vi "规范时间戳.vi"(11 "字符串":string) -> (3 "result string":string)   [LabVIEW 2016, in "数据传输系统-04.lvlib"]
panel:
  out "输出 1":timestamp
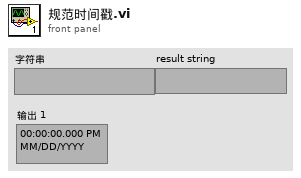
[diagram p1: front panel]
types:
  T1 = typedef "LVDateTimeRec.ctl" = cluster{"秒数的小数部分":dbl, "秒":i32, "分":i32, "时":i32, "日":i32, "月":i32, "年":i32, "天数（周）":i32, "天数（年）":i32, "DST":i32}
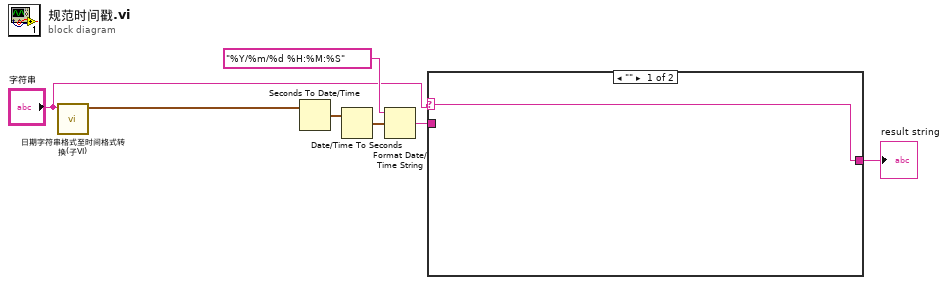
[diagram p0: block diagram]
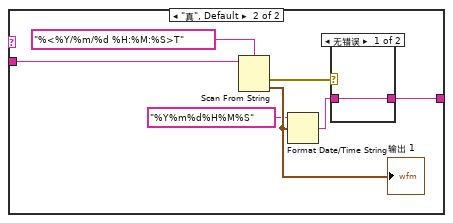
[diagram p2: hidden frame]
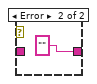
[diagram p3: hidden frame]
diagram:
  n1 = call "日期字符串格式至时间格式转换(子VI).vi"("data[0]"="字符串") -> ("time stamp"=w5:timestamp)  [unwired: 10 in]
  n2 = Seconds To Date/Time(time stamp (now)=w5) -> (date time rec=w6:T1)  [unwired: 1 in]
  n3 = Date/Time To Seconds(2:w6) -> (0:w4:timestamp)  [unwired: 1 in]
  n4 = Format Date/Time String(time format string (%c)="%Y/%m/%d %H:%M:%S" ("时间格式字符串(%c)"), seconds (now)=w4) -> (date/time string=w2:string)  [unwired: 1 in]
  n5 = case shown="\"\"" "字符串" {
    selector: "字符串" -> [w8 _]
    tunnel: w2 -> [_ w15]
    tunnel: [w8 w9] -> w7
    frame "" {
    }
    frame "真", Default {
      n6 = Scan From String(format string="%<%Y/%m/%d %H:%M:%S>T" ("格式字符串"), input string=w15) -> (error out=w11:errorcluster, output 1=w14:timestamp)  [unwired: 3 in, 2 out]
      "输出 1" <- w14
      n7 = Format Date/Time String(time format string (%c)="%Y%m%d%H%M%S" ("时间格式字符串(%c)"), seconds (now)=w14) -> (date/time string=w10:string)  [unwired: 1 in]
      n8 = case shown="无错误" w11 {
        tunnel: [w16 "" ("date/time string")] -> w9
        tunnel: w10 -> [w16 _]
        frame No Error {
        }
        frame Error {
        }
      }
    }
  }
  "result string" <- w7
